vi "Tosca-Save Session Info.vi"(0 "Session Info":T1={"Animal ID"="", "Session"=0, "Path"=path "", "Run"=1} {"Session" min=1 step=1}, 11 "error in (no error)":errorcluster) -> (15 "error out":errorcluster)   [LabVIEW 2020]
uses:
  Typedefs/Tosca-Session Info.ctl
  <vilib>/Utility/config.llb/Write Key (I32).vi
  <vilib>/Utility/config.llb/NI_LVConfig.lvlib
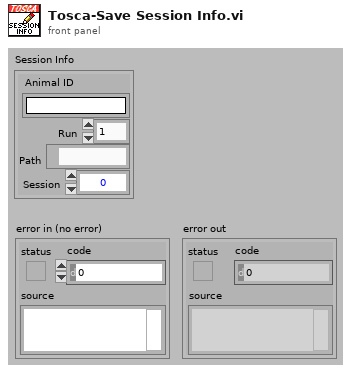
[diagram p1: front panel]
types:
  T1 = typedef "Tosca-Session Info.ctl" = cluster{"Animal ID":string, "Session":i32, "Path":path, "Run":i32}
  T2 = typedef "NI_LVConfig.lvlib/Config Data RefNum.ctl" = refnum<k1>
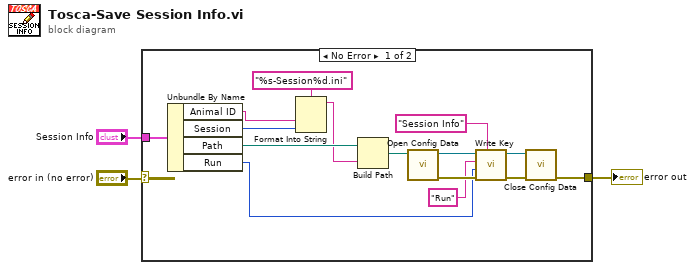
[diagram p0: block diagram]
diagram:
  n1 = case shown="No Error" "error in (no error)" {
    selector: "error in (no error)" -> [_ w19]
    tunnel: [w6 w19] -> w2
    tunnel: "Session Info" -> [w18 _]
    frame No Error {
      n2 = Unbundle By Name(w18) -> ("Animal ID"=w5:string, "Session"=w4:i32, "Path"=w16:path, "Run"=w10:i32)
      n3 = Format Into String(format string="%s-Session%d.ini", w5, w4) -> (resulting string=w15:string)  [unwired: 2 in, 1 out]
      n4 = Build Path(base path=w16, name or relative path=w15) -> (appended path=w14:path)
      n5 = call <vilib>:"Open Config Data.vi"("configuration file path"=w14) -> ("error out"=w13:errorcluster, "refnum"=w12:T2)  [unwired: 8 in, 1 out]
      n6 = call-poly <vilib>:"Write Key.vi"("section"="Session Info", "error in (no error)"=w13, "value"=w10, "key"="Run", "refnum"=w12) -> ("error out"=w8:errorcluster, "refnum out"=w7:T2)  [unwired: 4 in, 1 out]
      n7 = call <vilib>:"Close Config Data.vi"("error in (no error)"=w8, "refnum"=w7) -> ("error out"=w6:errorcluster)  [unwired: 8 in, 1 out]
    }
    frame Error {
    }
  }
  "error out" <- w2
